vi "all_values.vi"() -> ()   [LabVIEW 2018]
uses:
  <vilib>/Instr/_visa.llb/VISA Configure Serial Port (Instr).vi
panel:
  out "VISA resource name out":refnum<visa-resource-name>
  out "error out":errorcluster
  in  "unsigned byte array":u8[](array[numeric])
  in  "COM port":refnum<visa-resource-name>
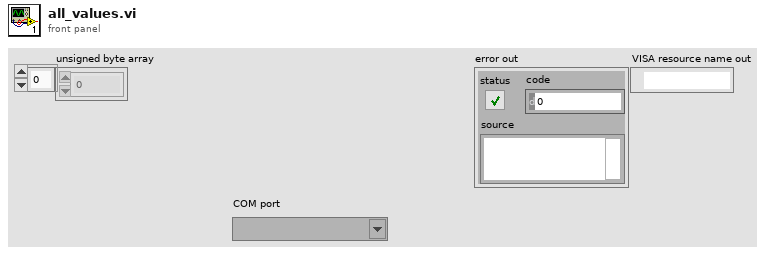
[diagram p1: front panel]
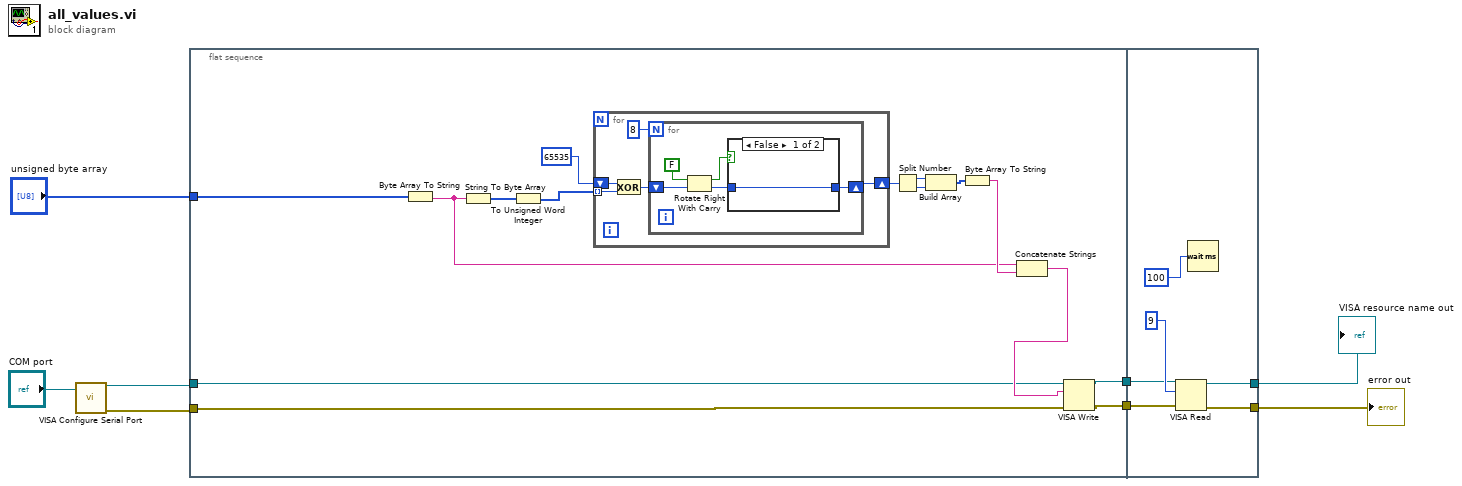
[diagram p0: block diagram]
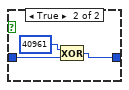
[diagram p2: hidden frame]
diagram:
  n1 = call-poly "VISA Configure Serial Port"("VISA resource name"="COM port") -> ("VISA resource name out"=w5:refnum<visa-resource-name>, "error out"=w4:errorcluster)  [unwired: 13 in]
  n2 = flat-sequence {
    tunnel: w5 -> [w13]
    tunnel: w4 -> [w12]
    tunnel: [w11] -> w8
    tunnel: [w10] -> w7
    tunnel: "unsigned byte array" -> [w9]
    tunnel: w8 -> [w41]
    tunnel: w7 -> [w40]
    tunnel: [w39] -> w1
    tunnel: [w38] -> w2
    frame #0 {
      n3 = Byte Array To String(unsigned byte array=w9) -> (string=w17:string)
      n4 = String To Byte Array(string=w17) -> (unsigned byte array=w21:u8[])
      n5 = To Unsigned Word Integer(number=w21) -> (unsigned 16bit integer=w22:u16[])
      n6 = for {
        shift-right: [w25] -> w23
        shift-left: u16 65535 -> [w26]
        tunnel: w22 -> [w24] mode=indexing
        n7 = Exclusive Or(1:w24, 2:w26) -> (0:w27:u16)
        n8 = for {
          N: 8 -> [_]
          shift-right: [w32] -> w25
          shift-left: w27 -> [w31]
          n9 = Rotate Right With Carry(2:w31, 3:FALSE ("Übertrag")) -> (0:w33:u16, 1:w30:bool)
          n10 = case shown="False" w30 {
            tunnel: w33 -> [w34 w36]
            tunnel: [w34 w35] -> w32
            frame False {
            }
            frame True {
              n11 = Exclusive Or(1:w36, 2:u16 40961) -> (0:w35:u16)
            }
          }
        }
      }
      n12 = Split Number(x=w23) -> (hi(x)=w20:u8, lo(x)=w19:u8)
      n13 = Build Array(w20, w19) -> (w16:u8[])
      n14 = Byte Array To String(unsigned byte array=w16) -> (string=w18:string)
      n15 = Concatenate Strings(w17, w18) -> (w14:string)
      n16 = VISA Write(VISA resource name=w13, write buffer=w14, error in (no error)=w12) -> (VISA resource name out=w11:refnum<visa-resource-name>, error out=w10:errorcluster)  [unwired: 1 out]
    }
    frame #1 {
      n17 = VISA Read(VISA resource name=w41, byte count=u32 9, error in (no error)=w40) -> (VISA resource name out=w39:refnum<visa-resource-name>, error out=w38:errorcluster)  [unwired: 2 out]
      n18 = Wait (ms)(milliseconds to wait=u32 100) -> ()  [unwired: 1 out]
    }
  }
  "error out" <- w2
  "VISA resource name out" <- w1
